vi "do_caxis_fit.vi"(8 "Error In":errorcluster, 10 "Sample":string, 11 "File Path":path) -> (0 "Error Out":errorcluster)   [LabVIEW 2019]
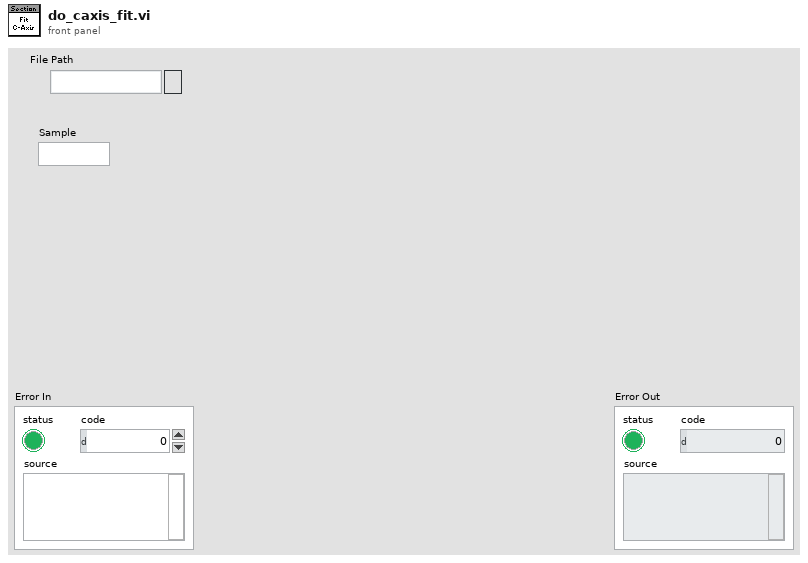
[diagram p1: front panel]
types:
  T1 = typedef "sample_results_cluster_typedef.ctl" = cluster{"File Path":string, "Sample":string, "Threshold":dbl, "Parameters":T2, "Writeable Parameters":T3, "Gain Results":T4[]}
  T2 = typedef "parameters_cluster_typedef.ctl" = cluster{"m1":dbl, "m2":dbl, "m3":dbl, "c":dbl, "D":dbl, "Beta":dbl, "center x":dbl, "center y":dbl}
  T3 = typedef "writeable_section_parameters_cluster_typedef.ctl" = cluster{"Section":string, "Method":i32, "Edge Mode":i32, "Grid Constant":i32, "Manual Sequence":i32, "ROI Size":i32, "Min Grain Size":dbl, "Comments":string, "File Path":string}
  T4 = typedef "grain_results_cluster_typedef.ctl" = cluster{"Grain Number":i32, "xi":dbl[], "phiin":dbl[], "Intensity":dbl[][], "Best Fit Intensity":dbl[][], "Best Fit Parameters":dbl[][], "Polarizer 1 Angle":dbl[][], "Polarizer 2 Angle":dbl[][], "Best Extinction Angle":dbl[], "Best Extinction Angle Corrected":dbl[], "Thetac":dbl, "Phic":dbl, "ROI":cluster{"Global Rectangle":i32[], "Contours":cluster{"Contour Type":u32, "ROI Type":u32, "Points":i32[]}[]}, "a":dbl, "b":dbl, "sequences available":dbl, "sequences used":dbl, "Contrast":dbl[], "Rsq":dbl}
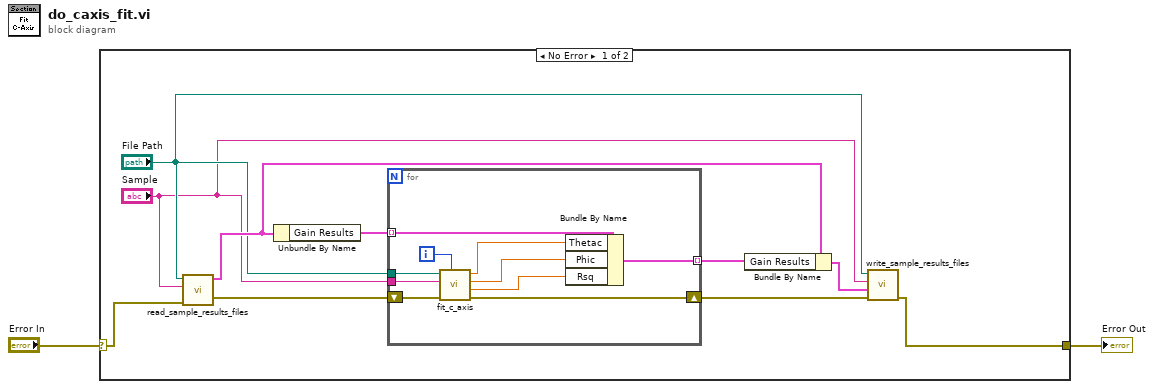
[diagram p0: block diagram]
diagram:
  n1 = case shown="No Error" "Error In" {
    selector: "Error In" -> [w12 w23]
    tunnel: [w3 w23] -> w1
    frame No Error {
      n2 = call "read_sample_results_files.vi"("Error In"=w12, "Sample"="Sample", "File Path"="File Path") -> ("Error Out"=w11:errorcluster, "Sample Results"=w9:T1)  [unwired: 7 in]
      n3 = Unbundle By Name(w9) -> ("Gain Results"=w10:T4[])
      n4 = for {
        tunnel: "File Path" -> [w22]
        tunnel: "Sample" -> [w21]
        tunnel: w10 -> [w18] mode=indexing
        tunnel: [w14] -> w8 mode=indexing
        shift-right: [w13] -> w7
        shift-left: w11 -> [w20]
        i -> [w19]
        n5 = call "fit_c_axis.vi"("Grain Number"=w19, "Error In"=w20, "Sample"=w21, "File Path Control"=w22) -> ("Error Out"=w13:errorcluster, "Best R2"=w15:dbl, "Phi min"=w16:dbl, "Theta min"=w17:dbl)  [unwired: 4 in]
        n6 = Bundle By Name(cluster=w18, "Thetac"=w17, "Phic"=w16, "Rsq"=w15) -> (w14:T4)
      }
      n7 = Bundle By Name(cluster=w9, "Gain Results"=w8) -> (w4:T1)
      n8 = call "write_sample_results_files.vi"("Error In"=w7, "Sample Results"=w4, "Sample"="Sample", "File Path"="File Path") -> ("Error Out"=w3:errorcluster)  [unwired: 7 in]
    }
    frame Error {
    }
  }
  "Error Out" <- w1
